vi "Run Filter.vi"(8 "error in (no error)":errorcluster, 10 "resource entries in":T1(array[cluster]) {"FPGA CD Ref" format="%.0x"; "reserver" format="%.0x"}, 11 "And Filter in":refnum<class "AND Filter.lvclass">) -> (0 "error out":errorcluster, 2 "resource entries out":T1(array[cluster]) {"FPGA CD Ref" format="%.0x"; "reserver" format="%.0x"})   [LabVIEW 2016, in "FPGA Resource Manager.lvlib" / "AND Filter.lvclass"]
uses:
  FPGA RM Test Client Configuration.llb/AND Filter.lvclass
  FPGA RM Test Client Configuration.llb/AND Filter.lvclass/AND Filter.ctl
  FPGA RM Test Client Configuration.llb/Filter.lvclass
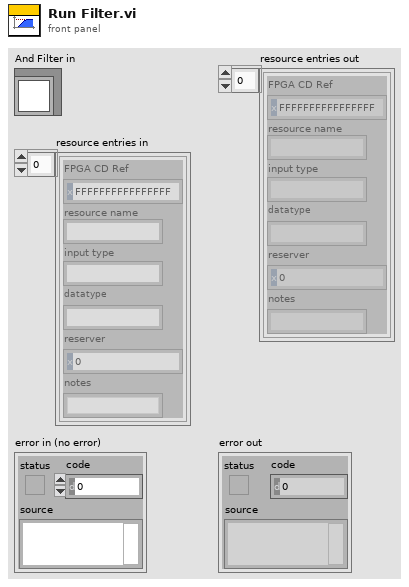
[diagram p1: front panel]
types:
  T1 = cluster{"FPGA CD Ref":u64, "resource name":string, "input type":string, "datatype":string, "reserver":u64, "notes":string}[]
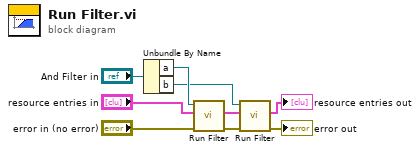
[diagram p0: block diagram]
diagram:
  n1 = Unbundle By Name("And Filter in") -> ("a"=w8:refnum<class "Filter.lvclass">, "b"=w6:refnum<class "Filter.lvclass">)
  n2 = call-dynamic "Run Filter.vi"("error in (no error)"="error in (no error)", "resource entries in"="resource entries in", "Filter in"=w8) -> ("error out"=w4:errorcluster, "resource entries out"=w5:T1)  [unwired: 7 in]
  n3 = call-dynamic "Run Filter.vi"("error in (no error)"=w4, "resource entries in"=w5, "Filter in"=w6) -> ("error out"=→"error out":errorcluster, "resource entries out"=→"resource entries out":T1)  [unwired: 7 in]
